vi "c.vi"   [LabVIEW 2020]
uses:
  b11eff79-1bba-4dac-99fe-af3bcc3b3ccb.vi
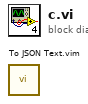
[diagram p0: block diagram]
diagram:
  n1 = call "To JSON Text.vim"() -> ()  [unwired: 10 in, 2 out]
